vi "FileFarsing.vi"() -> ()   [LabVIEW 2020]
panel:
  out "st1":string
  out "XY Graph":cluster{"array":dbl[], "array":dbl[]}[](graph)
  out "XY Graph 2":cluster{dbl[], dbl[]}[](graph)
  out "Array 7":dbl[](array[numeric])
  out "Array 6":dbl[](array[numeric])
  out "Array 5":dbl[](array[numeric])
  out "Array 4":dbl[](array[numeric])
  out "Array 3":T1(array[cluster])
  out "string array":string[](array[string])
  out "Array 2":T2(array[cluster])
  out "XXRMC":string
  out "time 2":string
  out "status":string
  out "lat 2":string
  out "NS 2":string
  out "lon 2":string
  out "EW 2":string
  out "spd":string
  out "cog":string
  out "data":string
  out "mv":string
  out "mv EW":string
  out "posMode":string
  out "navStatus":string
  out "cs":string
  out "Array":T3(array[cluster]) {"time" format="%^_9g"; "lat" format="%^#7.6g"}
  out "CS":string
  out "diffStation":string
  out "diffAge":string
  out "sep":string
  out "altUnit":string
  out "alt":string
  out "HDOP":string
  out "numSV":string
  out "quality":string
  out "EW":string
  out "lon":string
  out "NS":string
  out "lat":string
  out "time":string
  out "XXGGA":string
  out "size(s) 3":i32
  out "size(s) 2":i32
  out "size(s)":i32
  out "GPVTG":string[](array[string])
  out "GPRMC":string[](array[string])
  out "GPGAA":string[](array[string])
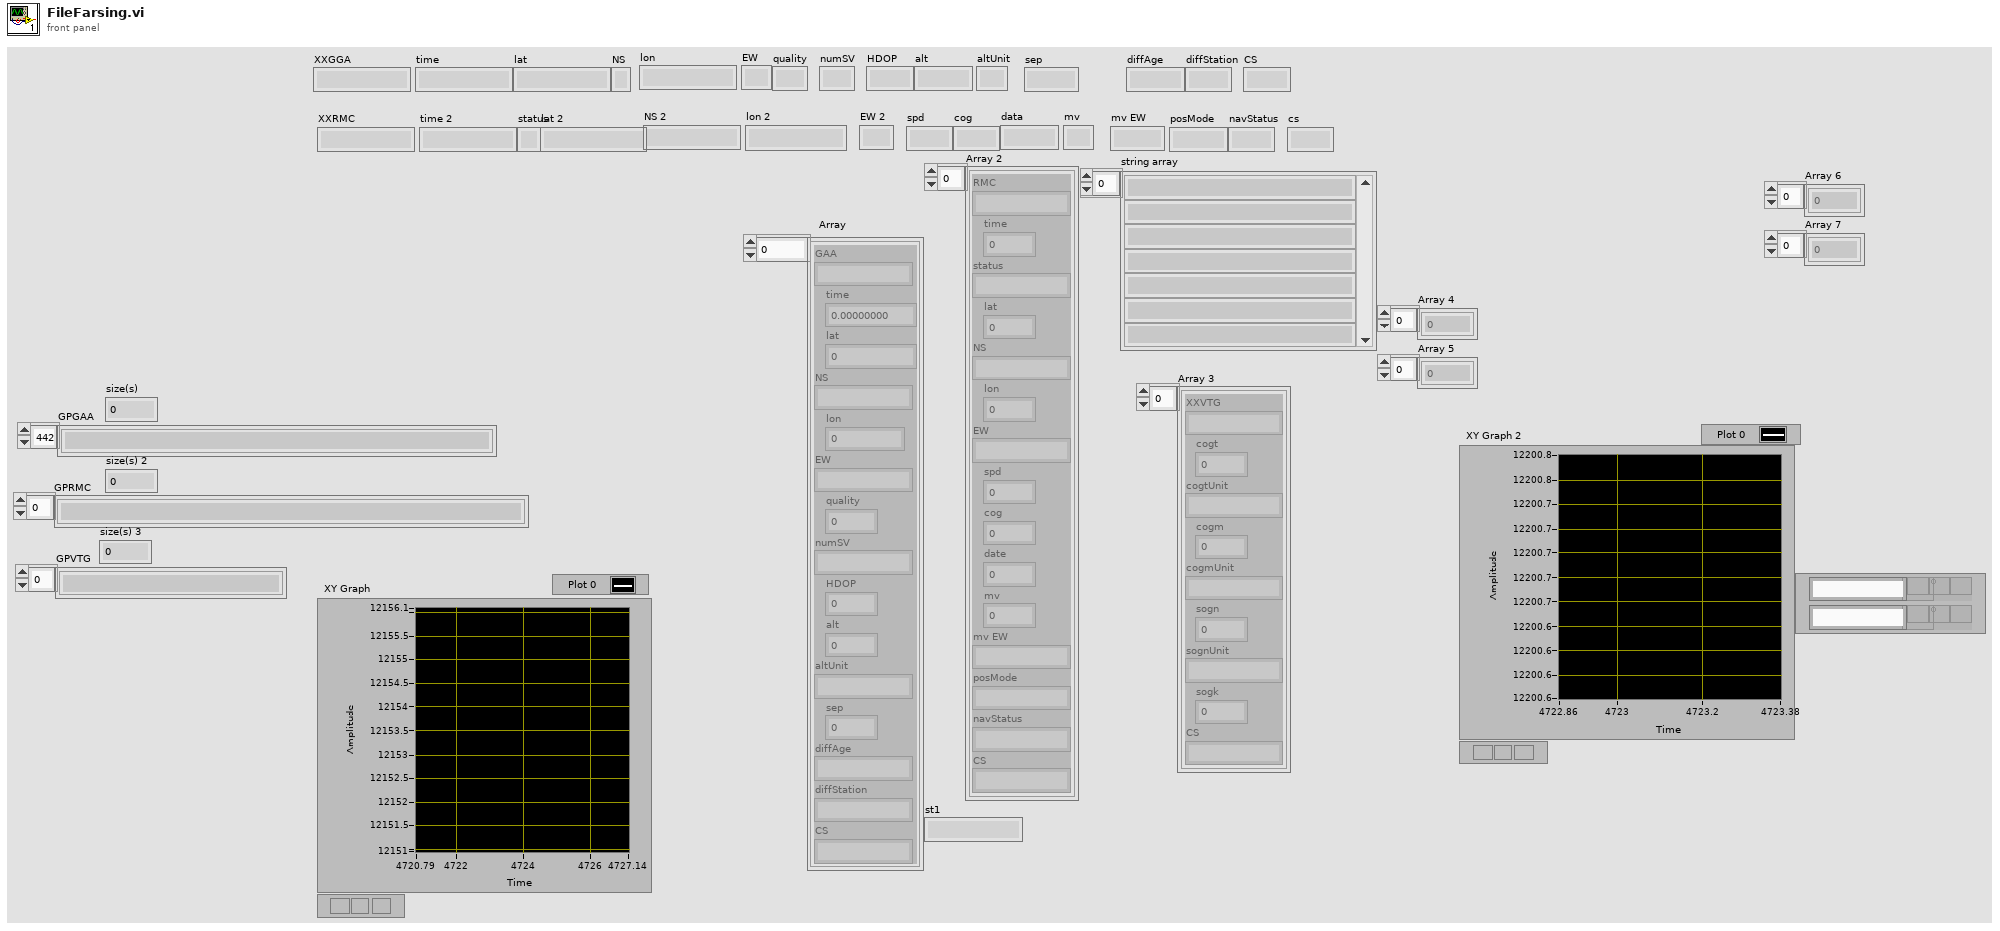
[diagram p1: front panel]
types:
  T1 = cluster{"XXVTG":string, "cogt":dbl, "cogtUnit":string, "cogm":dbl, "cogmUnit":string, "sogn":dbl, "sognUnit":string, "sogk":dbl, "CS":string}[]
  T2 = cluster{"RMC":string, "time":dbl, "status":string, "lat":dbl, "NS":string, "lon":dbl, "EW":string, "spd":dbl, "cog":dbl, "date":dbl, "mv":u16, "mv EW":string, "posMode":string, "navStatus":string, "CS":string}[]
  T3 = cluster{"GAA":string, "time":dbl, "lat":dbl, "NS":string, "lon":dbl, "EW":string, "quality":i32, "numSV":string, "HDOP":dbl, "alt":dbl, "altUnit":string, "sep":dbl, "diffAge":string, "diffStation":string, "CS":string}[]
  T4 = enum16{"open", "replace", "create", "open or create", "replace or create", "replace or create with confirmation"}
  T5 = cluster{"XXVTG":string, "cogt":dbl, "cogtUnit":string, "cogm":dbl, "cogmUnit":string, "sogn":dbl, "sognUnit":string, "sogk":dbl, "CS":string}
  T6 = cluster{"RMC":string, "time":dbl, "status":string, "lat":dbl, "NS":string, "lon":dbl, "EW":string, "spd":dbl, "cog":dbl, "date":dbl, "mv":u16, "mv EW":string, "posMode":string, "navStatus":string, "CS":string}
  T7 = cluster{"GAA":string, "time":dbl, "lat":dbl, "NS":string, "lon":dbl, "EW":string, "quality":i32, "numSV":string, "HDOP":dbl, "alt":dbl, "altUnit":string, "sep":dbl, "diffAge":string, "diffStation":string, "CS":string}
  T8 = cluster{"string array[0]":string, "string array[1]":string, "string array[2]":string, "string array[3]":string, "string array[4]":string, "string array[5]":string, "string array[6]":string, "string array[7]":string, "string array[8]":string}
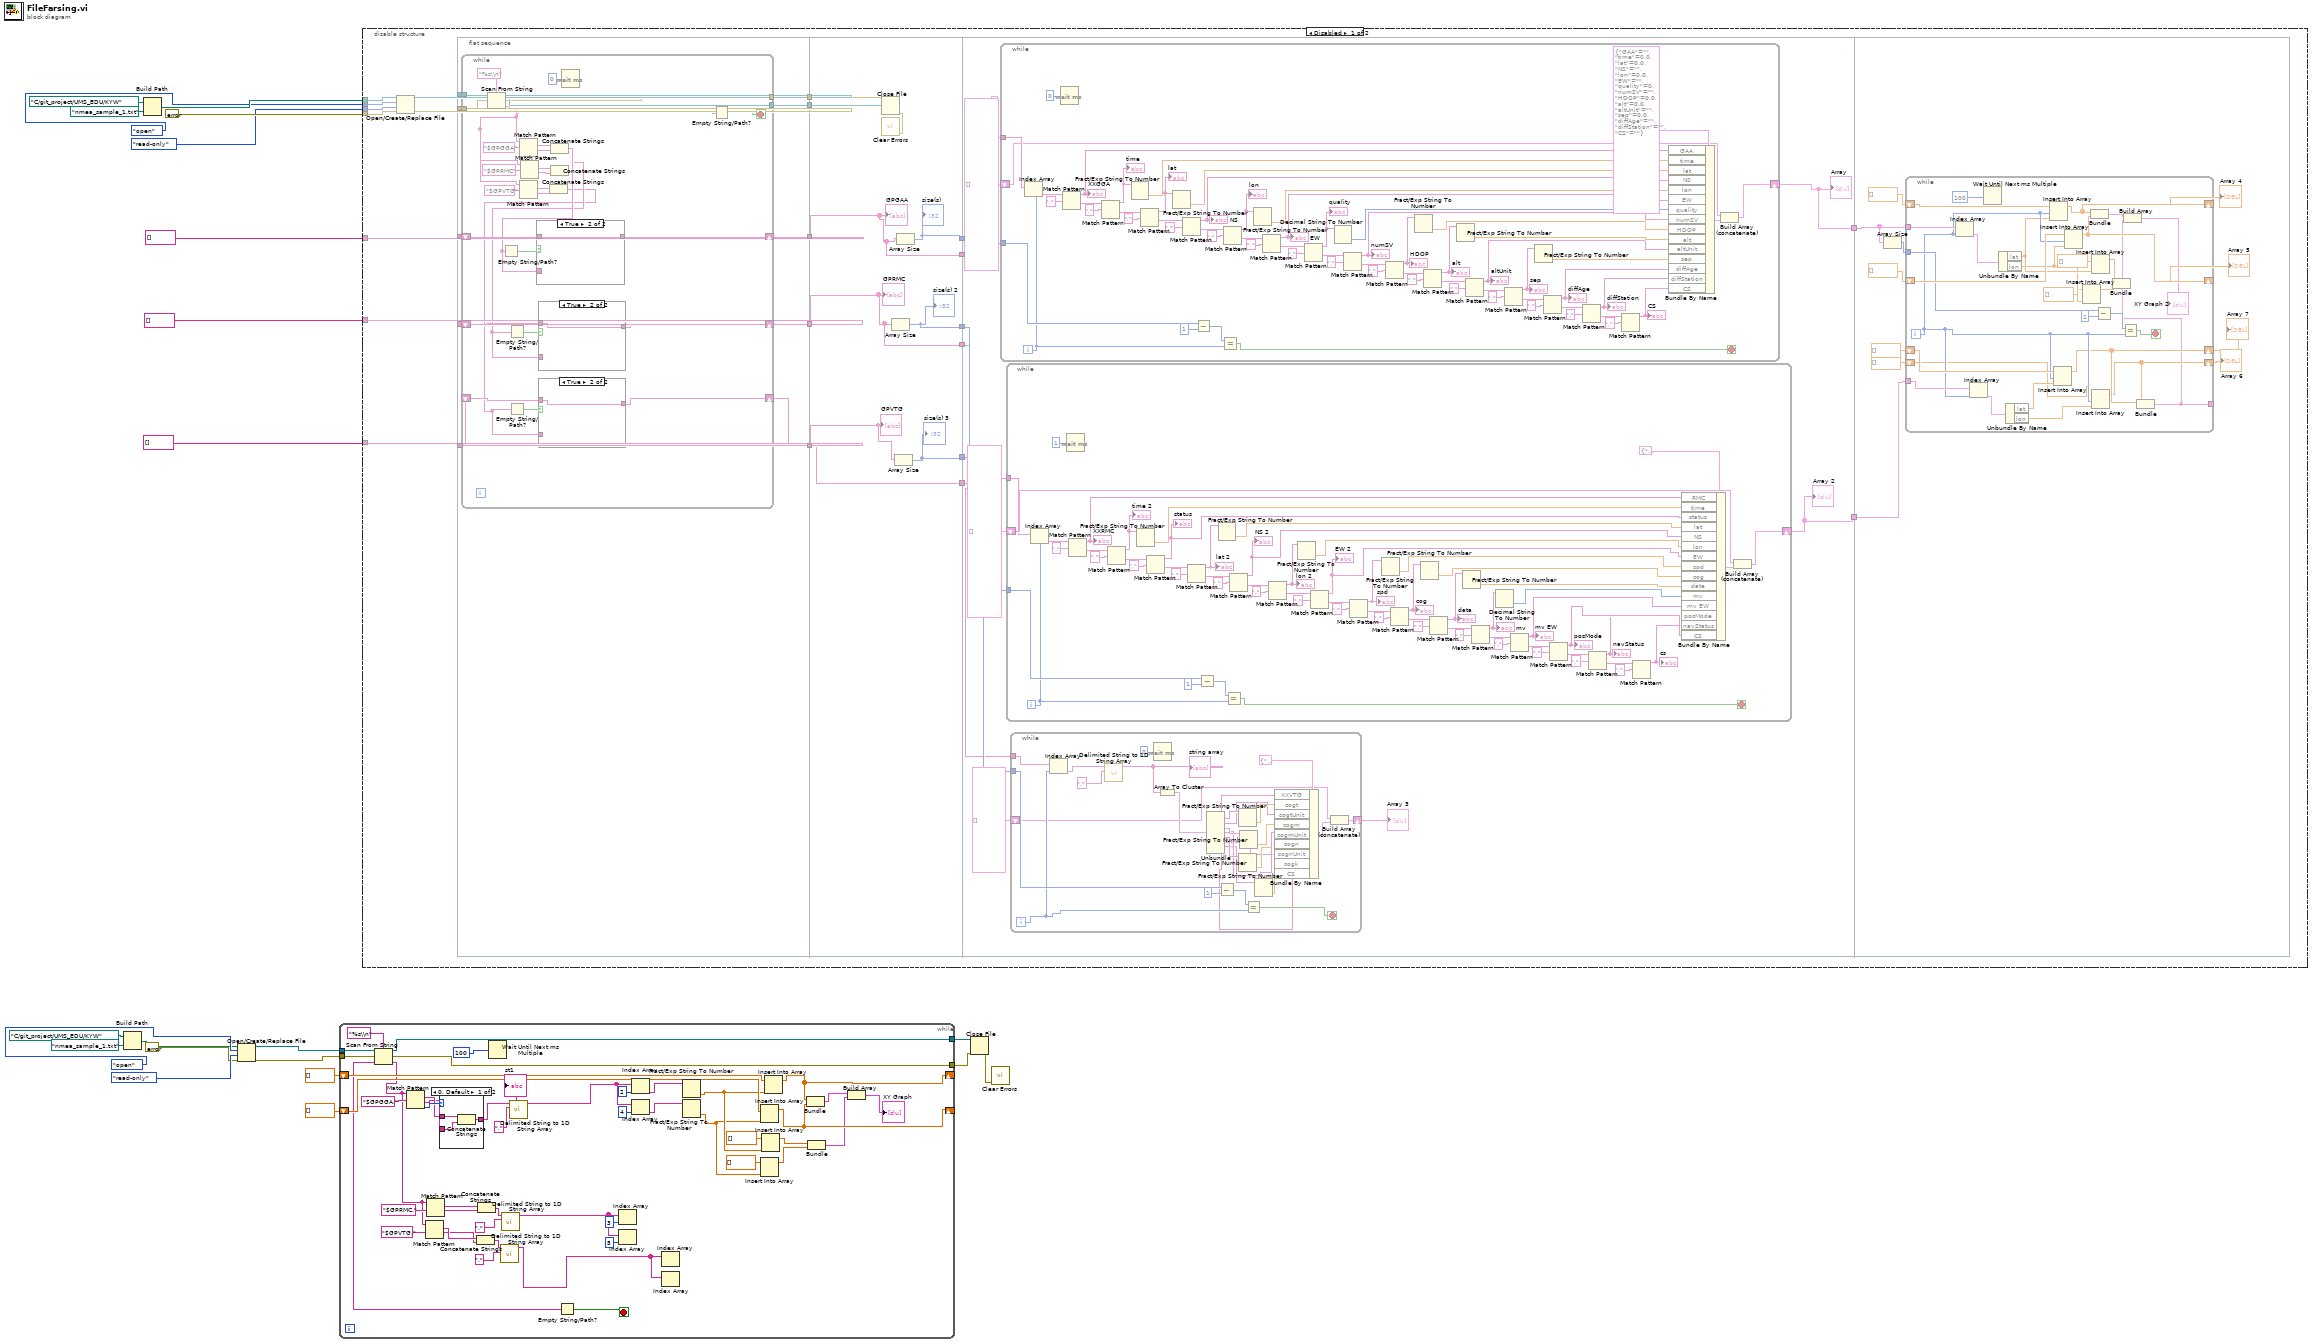
[diagram p0: block diagram]
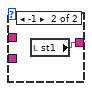
[diagram p2: hidden frame]
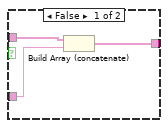
[diagram p3: hidden frame]
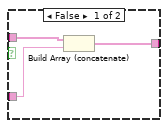
[diagram p4: hidden frame]
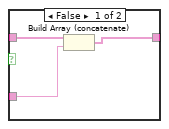
[diagram p5: hidden frame]
diagram:
  n1 = Build Path(base path=path "C:/git_project/UMS_EDU/KYW", name or relative path=path "nmea_sample_1.txt") -> (appended path=w8:path)
  n2 = Build Path(base path=path "C:/git_project/UMS_EDU/KYW", name or relative path=path "nmea_sample_1.txt") -> (appended path=w20:path)
  n3 = Open/Create/Replace File(file path (use dialog)=w8, error in=errorcluster {"status"=FALSE, "code"=0, "source"=""}, operation (0:open)=T4."open", access (0:read/write)=enum16{"read/write", "read-only", "write-only"}."read-only") -> (refnum out=w7:refnum<file>, error out=w6:errorcluster)  [unwired: 2 in, 1 out]
  n4 = while {
    tunnel: w7 -> [w68]
    tunnel: w6 -> [w67]
    tunnel: [w52] -> w5
    tunnel: [w51] -> w4
    shift-right: [w38] -> _
    shift-left: dbl[] [] -> [w40]
    shift-right: [w37] -> _
    shift-left: dbl[] [] -> [w39]
    stop <- w65 stop-if-true
    n5 = Scan From String("%s\\n" ("format string"), w68, w67) -> (w51:refnum<file>, w52:errorcluster, output 1=w23:string)  [unwired: 1 in]
    n6 = Match Pattern(string=w23, regular expression="$GPGGA,") -> (match substring=w26:string, after substring=w25:string, offset past match=w27:i32)  [unwired: 1 in, 1 out]
    n7 = Match Pattern(string=w23, regular expression="$GPVTG,") -> (match substring=w54:string, after substring=w53:string)  [unwired: 1 in, 2 out]
    n8 = Match Pattern(string=w23, regular expression="$GPRMC,") -> (match substring=w56:string, after substring=w55:string)  [unwired: 1 in, 2 out]
    n9 = case shown="0, Default" w27 {
      tunnel: w26 -> [w71 _]
      tunnel: w25 -> [w70 _]
      tunnel: [w69 w72] -> w24
      frame 0, Default {
        n10 = Concatenate Strings(w71, w70) -> (w69:string)
      }
      frame -1 {
        n11 = local read "st1"() -> (w72:string)
      }
    }
    "st1" <- w24
    n12 = Concatenate Strings(w54, w53) -> (w57:string)
    n13 = Concatenate Strings(w56, w55) -> (w59:string)
    n14 = Wait Until Next ms Multiple(millisecond multiple=u32 100 ("milliseconds to wait")) -> ()  [unwired: 1 out]
    n15 = call <vilib>:"Delimited String to 1D String Array.vi"("delimiter"=",", "delimited string"=w57) -> ("string array"=w48:string[])  [unwired: 9 in]
    n16 = call <vilib>:"Delimited String to 1D String Array.vi"("delimiter"=",", "delimited string"=w59) -> ("string array"=w49:string[])  [unwired: 9 in]
    n17 = call <vilib>:"Delimited String to 1D String Array.vi"("delimiter"=",", "delimited string"=w24) -> ("string array"=w50:string[])  [unwired: 9 in]
    n18 = Empty String/Path?(string/path=w23) -> (empty?=w65:bool)
    n19 = Index Array(array=w49, index=3) -> ()  [unwired: 1 out]
    n20 = Index Array(array=w49, index=5) -> ()  [unwired: 1 out]
    n21 = Index Array(array=w50, index=2) -> (element=w42:string)
    n22 = Index Array(array=w50, index=4) -> (element=w43:string)
    n23 = Index Array(array=w48) -> ()  [unwired: 1 in, 1 out]
    n24 = Index Array(array=w48) -> ()  [unwired: 1 in, 1 out]
    n25 = Fract/Exp String To Number(string=w42) -> (number=w34:dbl)  [unwired: 3 in, 1 out]
    n26 = Fract/Exp String To Number(string=w43) -> (number=w33:dbl)  [unwired: 3 in, 1 out]
    n27 = Insert Into Array(array=w39, new element=w33) -> (w37:dbl[])  [unwired: 1 in]
    n28 = Insert Into Array(array=dbl[] [], new element=w33) -> (w32:dbl[])  [unwired: 1 in]
    n29 = Insert Into Array(array=dbl[] [], new element=w34) -> (w31:dbl[])  [unwired: 1 in]
    n30 = Insert Into Array(array=w40, new element=w34) -> (w38:dbl[])  [unwired: 1 in]
    n31 = Bundle(w38, w37) -> (w29:cluster{dbl[], dbl[]})  [unwired: 1 in]
    n32 = Bundle("array"=w31, "array"=w32) -> (w30:cluster{"array":dbl[], "array":dbl[]})  [unwired: 1 in]
    n33 = Build Array(w29, w30) -> (→"XY Graph":cluster{"array":dbl[], "array":dbl[]}[])
  }
  n34 = disable-structure shown="Disabled" {
    disable-tunnel: w20 -> [w81 _]
    disable-tunnel: errorcluster {"status"=FALSE, "code"=0, "source"=""} ("error in") -> [w80 _]
    disable-tunnel: T4."open" ("operation (0:open)") -> [w79 _]
    disable-tunnel: enum16{"read/write", "read-only", "write-only"}."read-only" ("access (0:read/write)") -> [w78 _]
    disable-tunnel: string[] [] -> [w75 _]
    disable-tunnel: string[] [] -> [w74 _]
    disable-tunnel: string[] [] -> [w73 _]
    frame Disabled {
      n35 = Open/Create/Replace File(file path (use dialog)=w81, error in=w80, operation (0:open)=w79, access (0:read/write)=w78) -> (refnum out=w77:refnum<file>, error out=w76:errorcluster)  [unwired: 2 in, 1 out]
      n36 = flat-sequence {
        tunnel: w77 -> [w103]
        tunnel: w76 -> [w102]
        tunnel: w75 -> [w100]
        tunnel: w74 -> [w98]
        tunnel: w73 -> [w97]
        tunnel: [w104] -> w94
        tunnel: [w101] -> w93
        tunnel: [w99] -> w92
        tunnel: [w96] -> w91
        tunnel: [w95] -> w90
        tunnel: w94 -> [w152]
        tunnel: w93 -> [w153]
        tunnel: w92 -> [w149]
        tunnel: w91 -> [w151]
        tunnel: w90 -> [w150]
        tunnel: [w151] -> w89
        tunnel: [w150] -> w88
        tunnel: [w149] -> w87
        tunnel: [w148] -> w86
        tunnel: [w147] -> w85
        tunnel: [w146] -> w84
        tunnel: w89 -> [w162]
        tunnel: w88 -> [w159]
        tunnel: w87 -> [w165]
        tunnel: w86 -> [w166]
        tunnel: w85 -> [w163]
        tunnel: w84 -> [w160]
        tunnel: [w156] -> w83
        tunnel: [w155] -> w82
        tunnel: w83 -> [w327]
        tunnel: w82 -> [w325]
        frame #0 {
          n37 = while {
            tunnel: [w121] -> w104
            tunnel: w103 -> [w123]
            tunnel: w102 -> [w122]
            tunnel: [w118] -> w101
            shift-right: [w115] -> w99
            shift-left: w100 -> [w116]
            shift-right: [w110] -> w96
            shift-left: w98 -> [w111]
            shift-right: [w107] -> w95
            shift-left: w97 -> [w108]
            stop <- w119 stop-if-true
            n38 = Scan From String("%s\\n" ("format string"), w123, w122) -> (w121:refnum<file>, w118:errorcluster, output 1=w120:string)  [unwired: 1 in]
            n39 = Match Pattern(string=w120, regular expression="$GPGGA") -> (match substring=w128:string, after substring=w129:string)  [unwired: 1 in, 2 out]
            n40 = Match Pattern(string=w120, regular expression="$GPVTG") -> (match substring=w125:string, after substring=w124:string)  [unwired: 1 in, 2 out]
            n41 = Match Pattern(string=w120, regular expression="$GPRMC") -> (match substring=w127:string, after substring=w126:string)  [unwired: 1 in, 2 out]
            n42 = Concatenate Strings(w125, w124) -> (w106:string)
            n43 = Empty String/Path?(string/path=w106) -> (empty?=w109:bool)
            n44 = case shown="True" w109 {
              tunnel: w106 -> [w136 _]
              tunnel: w108 -> [w135 w137]
              tunnel: [w134 w137] -> w107
              frame False {
                n45 = Build Array (concatenate)(w135, w136) -> (w134:string[])
              }
              frame True {
              }
            }
            n46 = Concatenate Strings(w128, w129) -> (w114:string)
            n47 = Empty String/Path?(string/path=w114) -> (empty?=w117:bool)
            n48 = case shown="True" w117 {
              tunnel: w116 -> [w144 w145]
              tunnel: [w143 w145] -> w115
              tunnel: w114 -> [w142 _]
              frame False {
                n49 = Build Array (concatenate)(w144, w142) -> (w143:string[])
              }
              frame True {
              }
            }
            n50 = Concatenate Strings(w127, w126) -> (w112:string)
            n51 = Empty String/Path?(string/path=w112) -> (empty?=w113:bool)
            n52 = case shown="True" w113 {
              tunnel: w112 -> [w140 _]
              tunnel: w111 -> [w139 w141]
              tunnel: [w138 w141] -> w110
              frame False {
                n53 = Build Array (concatenate)(w139, w140) -> (w138:string[])
              }
              frame True {
              }
            }
            n54 = Wait (ms)(milliseconds to wait=u32 0) -> ()  [unwired: 1 out]
            n55 = Empty String/Path?(string/path=w120) -> (empty?=w119:bool)
          }
        }
        frame #1 {
          n56 = Close File(refnum=w152, error in=w153) -> (error out=w154:errorcluster)  [unwired: 1 out]
          n57 = call <vilib>:"Clear Errors.vi"("error in (no error)"=w154) -> ()  [unwired: 5 in, 2 out]
          n58 = Array Size(array=w151) -> (size(s)=w147:i32)
          "size(s) 2" <- w147
          n59 = Array Size(array=w150) -> (size(s)=w146:i32)
          "size(s) 3" <- w146
          n60 = Array Size(array=w149) -> (size(s)=w148:i32)
          "size(s)" <- w148
          "GPGAA" <- w149
          "GPRMC" <- w151
          "GPVTG" <- w150
        }
        frame #2 {
          n61 = while {
            tunnel: w166 -> [w320]
            tunnel: w165 -> [w315]
            shift-right: [w283] -> w156
            shift-left: T3 [] -> [w258]
            i -> [w316]
            stop <- w317 stop-if-true
            n62 = Index Array(array=w315, index=w316) -> (element=w299:string)
            n63 = Wait (ms)(milliseconds to wait=u32 0) -> ()  [unwired: 1 out]
            n64 = Match Pattern(string=w299, regular expression=",") -> (before substring=w274:string, after substring=w298:string)  [unwired: 1 in, 2 out]
            "XXGGA" <- w274
            n65 = Match Pattern(string=w298, regular expression=",") -> (before substring=w281:string, after substring=w297:string)  [unwired: 1 in, 2 out]
            "time" <- w281
            n66 = Fract/Exp String To Number(string=w281) -> (number=w273:dbl)  [unwired: 3 in, 1 out]
            n67 = Match Pattern(string=w297, regular expression=",") -> (before substring=w282:string, after substring=w286:string)  [unwired: 1 in, 2 out]
            "lat" <- w282
            n68 = Fract/Exp String To Number(string=w282) -> (number=w272:dbl)  [unwired: 3 in, 1 out]
            n69 = Match Pattern(string=w286, regular expression=",") -> (before substring=w271:string, after substring=w285:string)  [unwired: 1 in, 2 out]
            "NS" <- w271
            n70 = Subtract(x=w320, y=1) -> (x-y=w318:i32)
            n71 = Equal?(x=w318, y=w316) -> (x = y?=w317:bool)
            n72 = Match Pattern(string=w285, regular expression=",") -> (before substring=w280:string, after substring=w284:string)  [unwired: 1 in, 2 out]
            "lon" <- w280
            n73 = Fract/Exp String To Number(string=w280) -> (number=w270:dbl)  [unwired: 3 in, 1 out]
            n74 = Match Pattern(string=w284, regular expression=",") -> (before substring=w269:string, after substring=w296:string)  [unwired: 1 in, 2 out]
            "EW" <- w269
            n75 = Match Pattern(string=w296, regular expression=",") -> (before substring=w279:string, after substring=w295:string)  [unwired: 1 in, 2 out]
            "quality" <- w279
            n76 = Decimal String To Number(string=w279) -> (number=w268:i32)  [unwired: 2 in, 1 out]
            n77 = Match Pattern(string=w295, regular expression=",") -> (before substring=w267:string, after substring=w293:string)  [unwired: 1 in, 2 out]
            "numSV" <- w267
            n78 = Match Pattern(string=w293, regular expression=",") -> (before substring=w278:string, after substring=w292:string)  [unwired: 1 in, 2 out]
            "HDOP" <- w278
            n79 = Fract/Exp String To Number(string=w278) -> (number=w266:dbl)  [unwired: 3 in, 1 out]
            n80 = Match Pattern(string=w292, regular expression=",") -> (before substring=w277:string, after substring=w291:string)  [unwired: 1 in, 2 out]
            "alt" <- w277
            n81 = Fract/Exp String To Number(string=w277) -> (number=w265:dbl)  [unwired: 3 in, 1 out]
            n82 = Match Pattern(string=w291, regular expression=",") -> (before substring=w264:string, after substring=w290:string)  [unwired: 1 in, 2 out]
            "altUnit" <- w264
            n83 = Match Pattern(string=w290, regular expression=",") -> (before substring=w276:string, after substring=w289:string)  [unwired: 1 in, 2 out]
            "sep" <- w276
            n84 = Fract/Exp String To Number(string=w276) -> (number=w263:dbl)  [unwired: 3 in, 1 out]
            n85 = Match Pattern(string=w289, regular expression=",") -> (before substring=w262:string, after substring=w288:string)  [unwired: 1 in, 2 out]
            "diffAge" <- w262
            n86 = Match Pattern(string=w288, regular expression=",") -> (before substring=w261:string, after substring=w287:string)  [unwired: 1 in, 2 out]
            "diffStation" <- w261
            n87 = Match Pattern(string=w287, regular expression=",") -> (before substring=w260:string)  [unwired: 1 in, 3 out]
            "CS" <- w260
            n88 = Bundle By Name(cluster=T7 {"GAA"="", "time"=0.0, "lat"=0.0, "NS"="", "lon"=0.0, "EW"="", "quality"=0, "numSV"="", "HDOP"=0.0, "alt"=0.0, "altUnit"="", "sep"=0.0, "diffAge"="", "diffStation"="", "CS"=""}, "GAA"=w274, "time"=w273, "lat"=w272, "NS"=w271, "lon"=w270, "EW"=w269, "quality"=w268, "numSV"=w267, "HDOP"=w266, "alt"=w265, "altUnit"=w264, "sep"=w263, "diffAge"=w262, "diffStation"=w261, "CS"=w260) -> (w259:T7)
            n89 = Build Array (concatenate)(w258, w259) -> (w283:T3)
          }
          "Array" <- w156
          n90 = while {
            tunnel: w163 -> [w257]
            shift-right: [w221] -> w155
            shift-left: T2 [] -> [w212]
            tunnel: w162 -> [w211]
            i -> [w253]
            stop <- w254 stop-if-true
            n91 = Index Array(array=w211, index=w253) -> (element=w237:string)
            n92 = Wait (ms)(milliseconds to wait=u32 1) -> ()  [unwired: 1 out]
            n93 = Match Pattern(string=w237, regular expression=",") -> (before substring=w217:string, after substring=w236:string)  [unwired: 1 in, 2 out]
            "XXRMC" <- w217
            n94 = Match Pattern(string=w236, regular expression=",") -> (before substring=w220:string, after substring=w235:string)  [unwired: 1 in, 2 out]
            "time 2" <- w220
            n95 = Fract/Exp String To Number(string=w220) -> (number=w216:dbl)  [unwired: 3 in, 1 out]
            n96 = Match Pattern(string=w235, regular expression=",") -> (before substring=w209:string, after substring=w224:string)  [unwired: 1 in, 2 out]
            "status" <- w209
            n97 = Match Pattern(string=w224, regular expression=",") -> (before substring=w208:string, after substring=w223:string)  [unwired: 1 in, 2 out]
            "lat 2" <- w208
            n98 = Subtract(x=w257, y=1) -> (x-y=w255:i32)
            n99 = Fract/Exp String To Number(string=w208) -> (number=w207:dbl)  [unwired: 3 in, 1 out]
            n100 = Equal?(x=w255, y=w253) -> (x = y?=w254:bool)
            n101 = Match Pattern(string=w223, regular expression=",") -> (before substring=w206:string, after substring=w222:string)  [unwired: 1 in, 2 out]
            "NS 2" <- w206
            n102 = Match Pattern(string=w222, regular expression=",") -> (before substring=w205:string, after substring=w234:string)  [unwired: 1 in, 2 out]
            "lon 2" <- w205
            n103 = Fract/Exp String To Number(string=w205) -> (number=w204:dbl)  [unwired: 3 in, 1 out]
            n104 = Match Pattern(string=w234, regular expression=",") -> (before substring=w203:string, after substring=w233:string)  [unwired: 1 in, 2 out]
            "EW 2" <- w203
            n105 = Match Pattern(string=w233, regular expression=",") -> (before substring=w202:string, after substring=w231:string)  [unwired: 1 in, 2 out]
            "spd" <- w202
            n106 = Fract/Exp String To Number(string=w202) -> (number=w201:dbl)  [unwired: 3 in, 1 out]
            n107 = Match Pattern(string=w231, regular expression=",") -> (before substring=w219:string, after substring=w230:string)  [unwired: 1 in, 2 out]
            "cog" <- w219
            n108 = Fract/Exp String To Number(string=w219) -> (number=w215:dbl)  [unwired: 3 in, 1 out]
            n109 = Match Pattern(string=w230, regular expression=",") -> (before substring=w218:string, after substring=w229:string)  [unwired: 1 in, 2 out]
            "data" <- w218
            n110 = Fract/Exp String To Number(string=w218) -> (number=w214:dbl)  [unwired: 3 in, 1 out]
            n111 = Match Pattern(string=w229, regular expression=",") -> (before substring=w200:string, after substring=w228:string)  [unwired: 1 in, 2 out]
            "mv" <- w200
            n112 = Decimal String To Number(string=w200) -> (number=w199:i32)  [unwired: 2 in, 1 out]
            n113 = Match Pattern(string=w228, regular expression=",") -> (before substring=w198:string, after substring=w227:string)  [unwired: 1 in, 2 out]
            "mv EW" <- w198
            n114 = Match Pattern(string=w227, regular expression=",") -> (before substring=w197:string, after substring=w226:string)  [unwired: 1 in, 2 out]
            "posMode" <- w197
            n115 = Match Pattern(string=w226, regular expression=",") -> (before substring=w196:string, after substring=w225:string)  [unwired: 1 in, 2 out]
            "navStatus" <- w196
            n116 = Match Pattern(string=w225, regular expression=",") -> (before substring=w195:string)  [unwired: 1 in, 3 out]
            "cs" <- w195
            n117 = Bundle By Name(cluster=T6 {"RMC"="", "time"=0.0, "status"="", "lat"=0.0, "NS"="", "lon"=0.0, "EW"="", "spd"=0.0, "cog"=0.0, "date"=0.0, "mv"=0, "mv EW"="", "posMode"="", "navStatus"="", "CS"=""}, "RMC"=w217, "time"=w216, "status"=w209, "lat"=w207, "NS"=w206, "lon"=w204, "EW"=w203, "spd"=w201, "cog"=w215, "date"=w214, "mv"=w199, "mv EW"=w198, "posMode"=w196, "navStatus"=w195, "CS"=w197) -> (w213:T6)
            n118 = Build Array (concatenate)(w212, w213) -> (w221:T2)
          }
          "Array 2" <- w155
          n119 = while {
            tunnel: w160 -> [w191]
            tunnel: w159 -> [w190]
            shift-right: [w168] -> w158
            shift-left: T1 [] -> [w167]
            i -> [w189]
            stop <- w192 stop-if-true
            n120 = Index Array(array=w190, index=w189) -> (element=w188:string)
            n121 = call <vilib>:"Delimited String to 1D String Array.vi"("delimiter"="," ("regular expression"), "delimited string"=w188) -> ("string array"=w185:string[])  [unwired: 9 in]
            "string array" <- w185
            n122 = Wait (ms)(milliseconds to wait=u32 0) -> ()  [unwired: 1 out]
            n123 = Array To Cluster(array=w185) -> (cluster=w184:T8)
            n124 = Unbundle(w184) -> ("string array[0]"=w180:string, "string array[1]"=w183:string, "string array[2]"=w178:string, "string array[3]"=w182:string, "string array[4]"=w176:string, "string array[5]"=w181:string, "string array[6]"=w172:string, "string array[7]"=w171:string, "string array[8]"=w170:string)
            n125 = Subtract(x=w191, y=1) -> (x-y=w193:i32)
            n126 = Fract/Exp String To Number(string=w183) -> (number=w179:dbl)  [unwired: 3 in, 1 out]
            n127 = Fract/Exp String To Number(string=w181) -> (number=w175:dbl)  [unwired: 3 in, 1 out]
            n128 = Fract/Exp String To Number(string=w182) -> (number=w177:dbl)  [unwired: 3 in, 1 out]
            n129 = Equal?(x=w193, y=w189) -> (x = y?=w192:bool)
            n130 = Fract/Exp String To Number(string=w171) -> (number=w173:dbl)  [unwired: 3 in, 1 out]
            n131 = Bundle By Name(cluster=T5 {"XXVTG"="", "cogt"=0.0, "cogtUnit"="", "cogm"=0.0, "cogmUnit"="", "sogn"=0.0, "sognUnit"="", "sogk"=0.0, "CS"=""}, "XXVTG"=w180, "cogt"=w179, "cogtUnit"=w178, "cogm"=w177, "cogmUnit"=w176, "sogn"=w175, "sognUnit"=w172, "sogk"=w173, "CS"=w170) -> (w169:T5)
            n132 = Build Array (concatenate)(w167, w169) -> (w168:T1)
          }
          "Array 3" <- w158
        }
        frame #3 {
          n133 = Array Size(array=w327) -> (size(s)=w326:i32)
          n134 = while {
            tunnel: w327 -> [w360]
            shift-right: [w357] -> w330
            shift-left: dbl[] [] -> [w358]
            shift-right: [w355] -> w329
            shift-left: dbl[] [] -> [w356]
            tunnel: w326 -> [w352]
            tunnel: w325 -> [w349]
            shift-right: [w342] -> w323
            shift-left: dbl[] [] -> [w347]
            shift-right: [w341] -> w324
            shift-left: dbl[] [] -> [w343]
            tunnel: [w332] -> _
            i -> [w344]
            stop <- w351 stop-if-true
            n135 = Index Array(array=w360, index=w344) -> (element=w359:T7)
            n136 = Index Array(array=w349, index=w344) -> (element=w348:T6)
            n137 = Wait Until Next ms Multiple(millisecond multiple=u32 100 ("milliseconds to wait")) -> ()  [unwired: 1 out]
            n138 = Unbundle By Name(w359) -> ("lat"=w339:dbl, "lon"=w338:dbl)
            n139 = Unbundle By Name(w348) -> ("lat"=w346:dbl, "lon"=w345:dbl)
            n140 = Insert Into Array(array=w358, index=w344, new element=w339) -> (w357:dbl[])
            n141 = Insert Into Array(array=w347, index=w344, new element=w346) -> (w342:dbl[])
            n142 = Insert Into Array(array=w356, index=w344, new element=w338) -> (w355:dbl[])
            n143 = Insert Into Array(array=dbl[] [], new element=w338) -> (w334:dbl[])  [unwired: 1 in]
            n144 = Bundle(w357, w355) -> (w340:cluster{dbl[], dbl[]})  [unwired: 1 in]
            n145 = Insert Into Array(array=dbl[] [], new element=w339) -> (w335:dbl[])  [unwired: 1 in]
            n146 = Insert Into Array(array=w343, index=w344, new element=w345) -> (w341:dbl[])
            n147 = Subtract(x=w352, y=1) -> (x-y=w353:i32)
            n148 = Bundle("array"=w335, "array"=w334) -> ()  [unwired: 1 in, 1 out]
            n149 = Equal?(x=w353, y=w344) -> (x = y?=w351:bool)
            n150 = Bundle(w342, w341) -> (w332:cluster{dbl[], dbl[]})  [unwired: 1 in]
            n151 = Build Array(w340, w332) -> (→"XY Graph 2":cluster{dbl[], dbl[]}[])
          }
          "Array 4" <- w330
          "Array 5" <- w329
          "Array 6" <- w324
          "Array 7" <- w323
        }
      }
    }
    frame Enabled {
    }
  }
  n152 = Close File(refnum=w4, error in=w5) -> (error out=w3:errorcluster)  [unwired: 1 out]
  n153 = call <vilib>:"Clear Errors.vi"("error in (no error)"=w3) -> ()  [unwired: 5 in, 2 out]
